vi "GetSomethingByDate.vi"(8 "error in (no error)":errorcluster, 10 "Parámetro":T1, 11 "Time Stamp":timestamp format="%<%d/%m/%Y %I:%M:%S %p>T") -> (0 "error out":errorcluster, 3 "Result Set":dbl[](array[numeric]))   [LabVIEW 2020]
uses:
  Parametros.ctl
  <vilib>/drjdpowell/SQLite Library/SQL Connection/Open (path).vi
  <vilib>/drjdpowell/SQLite Library/SQL Connection/Open (string).vi
  <vilib>/AdvancedString/Path To Command Line String.vi
  <vilib>/drjdpowell/SQLite Library/SQL Connection/Execute SQL (1D DBL results).vi
  <vilib>/drjdpowell/SQLite Library/SQL Connection/Connection.lvclass
  <vilib>/drjdpowell/SQLite Library/SQLite.lvlib
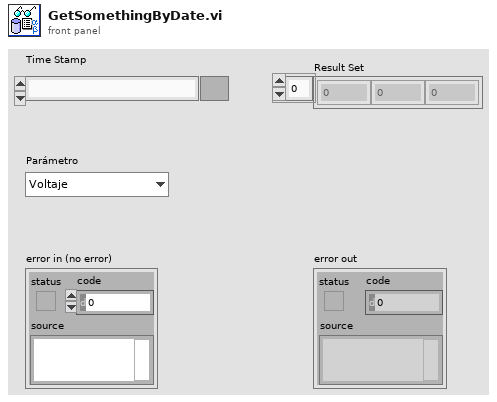
[diagram p1: front panel]
types:
  T1 = typedef "Parametros.ctl" = enum16{"Voltaje", "Corriente", "Temperatura de la carcasa", "Temperatura de balero", "Factor de potencia", "Velocidad de motor"}
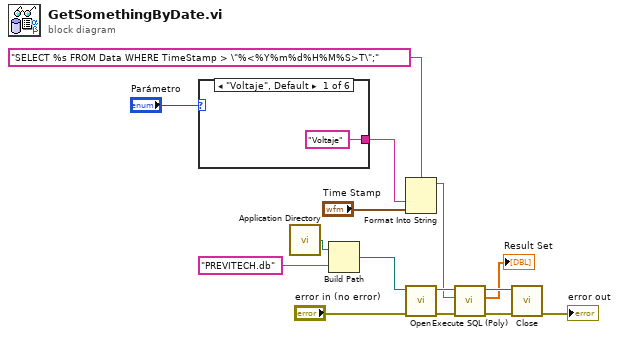
[diagram p0: block diagram]
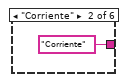
[diagram p2: hidden frame]
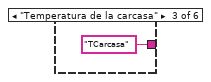
[diagram p3: hidden frame]
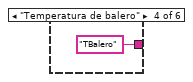
[diagram p4: hidden frame]
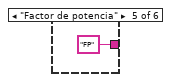
[diagram p5: hidden frame]
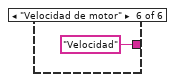
[diagram p6: hidden frame]
diagram:
  n1 = case shown="\"Voltaje\", Default" "Parámetro" {
    tunnel: ["Voltaje" "Corriente" "TCarcasa" "TBalero" "FP" "Velocidad"] -> w3
    frame "Voltaje", Default {
    }
    frame "Corriente" {
    }
    frame "Temperatura de la carcasa" {
    }
    frame "Temperatura de balero" {
    }
    frame "Factor de potencia" {
    }
    frame "Velocidad de motor" {
    }
  }
  n2 = call <vilib>:"Application Directory.vi"() -> ("Application Directory"=w15:path)
  n3 = Build Path(base path=w15, name or relative path="PREVITECH.db") -> (appended path=w13:path)
  n4 = Format Into String(format string="SELECT %s FROM Data WHERE TimeStamp > \"%<%Y%m%d%H%M%S>T\";", w3, "Time Stamp") -> (resulting string=w10:string)  [unwired: 2 in, 1 out]
  n5 = call-poly <vilib>:"Open.vi"("error in (no error)"="error in (no error)", "db file"=w13) -> ("error out"=w7:errorcluster, "SQLite Connection"=w12:refnum<class "Connection.lvclass">)  [unwired: 8 in]
  n6 = call-poly <vilib>:"Execute SQL (Poly).vi"("error in (no error)"=w7, "SQL"=w10, "SQLite Connection in"=w12) -> ("error out"=w6:errorcluster, "Result Set"=→"Result Set":dbl[], "SQLite Connection"=w11:refnum<class "Connection.lvclass">)  [unwired: 5 in, 1 out]
  n7 = call-dynamic "Close.vi"("error in (no error)"=w6, "SQLite Connection in"=w11) -> ("error out"=→"error out":errorcluster)  [unwired: 9 in]
